vi "ThresholdLevelFinderNEW.vi"(6 "Initial Threshold":i32=300, 7 "Channel":u32=1, 8 "error in (no error)":errorcluster, 9 "id_in":i32, 10 "connection ID":refnum<k5>, 11 "VISA resource name":refnum<visa-resource-name>="Oscilloscope") -> (0 "error out":errorcluster, 1 "id_out":i32, 2 "connection ID out":refnum<k5>, 3 "VISA resource name out":refnum<visa-resource-name>="Oscilloscope", 4 "threshold out":i32=495)   [LabVIEW 2009]
uses:
  Sum_Abrilader/L0_Sum_Adder Folder/C/Program Files/National Instruments/LabVIEW 2012/instr.lib/Agilent 8000 Series/Public/Data/Low Level/Fetch Measurement (More).vi
  Sum_Abrilader/L0_Sum_Adder Folder/C/Program Files/National Instruments/LabVIEW 2012/instr.lib/Agilent 8000 Series/Agilent 8000 Series.lvlib
panel:
  in  "increment":i32=20
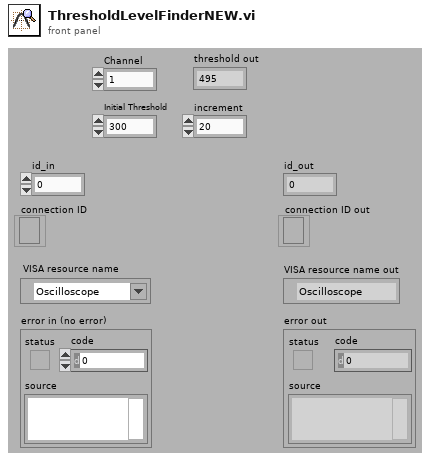
[diagram p1: front panel]
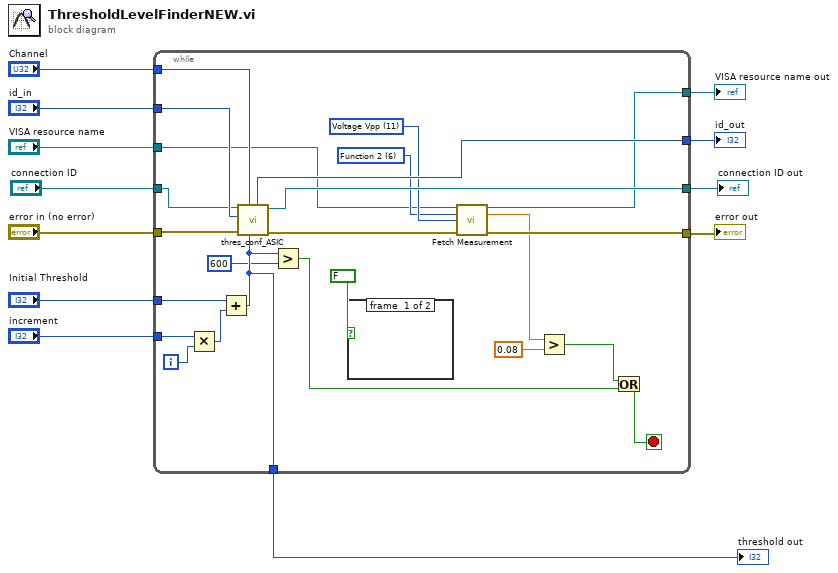
[diagram p0: block diagram]
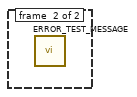
[diagram p2: hidden frame]
diagram:
  n1 = while {
    tunnel: "VISA resource name" -> [w20]
    tunnel: [w19] -> w11
    tunnel: "connection ID" -> [w25]
    tunnel: [w36] -> w9
    tunnel: "error in (no error)" -> [w24]
    tunnel: "id_in" -> [w32]
    tunnel: [w31] -> w6
    tunnel: "Channel" -> [w30]
    tunnel: [w27] -> w4
    tunnel: "Initial Threshold" -> [w29]
    tunnel: "increment" -> [w28]
    tunnel: [w18] -> w1
    i -> [w34]
    stop <- w16 stop-if-true
    w23 = 11 items=["Rise Time", "Fall Time", "Frequency", "Period", "Voltage RMS(AC)", "Voltage RMS(DC)", "Voltage RMS (AC,cycle)", "Voltage RMS (DC,cycle)", "Voltage Max", "Voltage Min", "Voltage Middle", "Voltage Vpp", "Voltage High", "Voltage Low", "Voltage Average", "Voltage Average (cycle)", "Width Negative", "Width Positive", "Duty Cycle Positive", "Amplitude", "Overshoot", "Preshoot", "Voltage Base", "Voltage Upper", "Time Max", "Time Min", "Color Grade Crossing", "Color Grade Eye Width", "Color Grade Eye Height", "Color Grade Eye Q-Factory", "Color Grade Eye Duty Cycle Distortion(Percent)", "Color Grade Eye Duty Cycle Distortion(Time)", "Color Grade Eye Jitter(PP)", "Color Grade Eye Width(RMS)", "Cycle-cycle Duty Jitter(Rising)", "Cycle-cycle Duty Jitter(Falling)", "Cycle-cycle Jitter(Rising)", "Cycle-cycle Jitter(Falling)", "Cycle-cycle - Width", "Cycle-cycle + Width", "Date Rate", "Unit Interval", "FFT Delta Frequency", "FFT Delta Magnitude", "FFT Frequency", "FFT Magnitude", "Slew Rate", "Area (Entire Display)", "Area(Single Cycle)", "Duty Cycle (Rising)", "Duty Cycle (Falling)"] ("Measurement Function (0: Rise Time)")
    w22 = 6 items=["Channel 1"=1, "Channel 2"=2, "Channel 3"=3, "Channel 4"=4, "Function 1"=5, "Function 2"=6, "Function 3"=7, "Function 4"=8, "Memory 1"=9, "Memory 2"=10, "Memory 3"=11, "Memory 4"=12] ("Channel (1: Channel 1)")
    n2 = Multiply(x=w28, y=w34) -> (x*y=w33:i32)
    n3 = Add(x=w29, y=w33) -> (x+y=w27:i32)
    n4 = call "thres_conf_ASIC.vi"("threshold"=w27, "Ring"=w30, "error out 3"=w24, "Id in"=w32, "connection ID"=w25) -> ("error out 2"=w21:errorcluster, "connection ID out"=w36:refnum<k5>, "Id out"=w31:i32)  [unwired: 3 in, 1 out]
    n5 = Greater?(x=w27, y=600) -> (0:w14:bool)
    n6 = case shown="True" FALSE {
      frame #0 {
      }
      frame #1 {
        n7 = call "ERROR_TEST_MESSAGE.vi"() -> ()  [unwired: 11 in, 1 out]
      }
    }
    n8 = call-poly "Fetch Measurement.vi"("VISA resource name"=w20, "Channel (1: Channel 1)"=w22, "Measurement Function (0: Rise Time)"=w23, "error in (no error)"=w21) -> ("VISA resource name out"=w19:refnum<visa-resource-name>, "Measurement"=w17:dbl, "error out"=w18:errorcluster)  [unwired: 9 in]
    n9 = Greater?(x=w17, y=0.08) -> (0:w15:bool)
    n10 = Or(x=w15, y=w14) -> (x .or. y?=w16:bool)
  }
  "VISA resource name out" <- w11
  "error out" <- w1
  "connection ID out" <- w9
  "id_out" <- w6
  "threshold out" <- w4
